vi "Put Signal over Mdsip Connection.vi"() -> ()   [LabVIEW 2015]
uses:
  Library/MDSplus.lvlib
panel:
  in  "Time":string
  in  "Data":string
  in  "Path":string
  in  "Shot":i32
  in  "Tree":string
  in  "IP:port":string
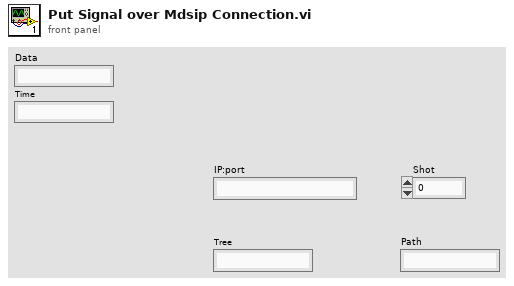
[diagram p1: front panel]
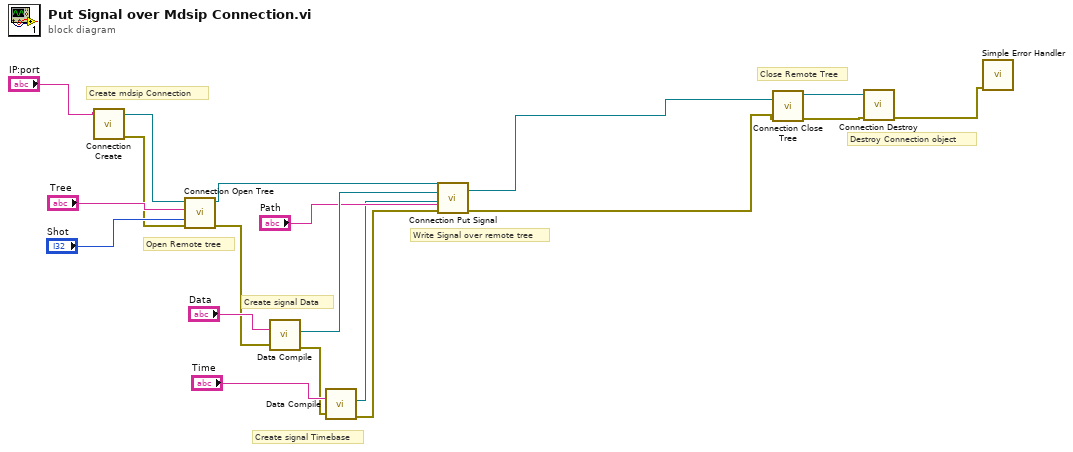
[diagram p0: block diagram]
diagram:
  # "Create signal Timebase"
  # "Create signal Data"
  # "Destroy Connection object"
  # "Close Remote Tree"
  # "Write Signal over remote tree"
  # "Open Remote tree"
  # "Create mdsip Connection"
  n1 = call "Connection Create.vi"("Ip : port"="IP:port") -> ("error out"=w12:errorcluster, "Connection DVR out"=w18:refnum<data-value>)  [unwired: 9 in]
  n2 = call "Connection Open Tree.vi"("error in (no error)"=w12, "Shot"="Shot", "Tree"="Tree", "Connection DVR in"=w18) -> ("error out"=w8:errorcluster, "Connection DVR out"=w1:refnum<data-value>)  [unwired: 6 in]
  n3 = call "Data Compile.vi"("error in (no error)"=w8, "Expression"="Data") -> ("error out"=w5:errorcluster, "Data out"=w7:refnum<data-value>)  [unwired: 7 in, 1 out]
  n4 = call "Data Compile.vi"("error in (no error)"=w5, "Expression"="Time") -> ("error out"=w4:errorcluster, "Data out"=w2:refnum<data-value>)  [unwired: 7 in, 1 out]
  n5 = call "Connection Put Signal.vi"("Connection DVR in"=w1, "Data"=w7, "time"=w2, "Path in"="Path", "error in (no error)"=w4) -> ("Connection DVR out"=w11:refnum<data-value>, "error out"=w10:errorcluster)  [unwired: 9 in]
  n6 = call "Connection Close Tree.vi"("error in (no error)"=w10, "Connection DVR in"=w11) -> ("error out"=w13:errorcluster, "Connection DVR out"=w14:refnum<data-value>)  [unwired: 8 in]
  n7 = call "Connection Destroy.vi"("error in (no error)"=w13, "Connection DVR in"=w14) -> ("error out"=w15:errorcluster)  [unwired: 9 in]
  n8 = call <vilib>:"Simple Error Handler.vi"("error in (no error)"=w15) -> ()  [unwired: 4 in, 5 out]
